vi "CREAR_BANDEJA_xml.vi"(0 "largo":u32, 1 "nombre bandeja":string, 2 "Nº de filas":u32, 3 "Nº de columnas":u32, 4 "Paso X":dbl, 5 "error in (no error)":errorcluster, 6 "path":path, 7 "Paso Y":dbl, 9 "DISTANCIA SUELO A CHIP":dbl, 10 "ancho":u32, 11 "Dist. borde bandeja a centro chip":dbl) -> (19 "error out":errorcluster)   [LabVIEW 2019]
uses:
  <vilib>/Utility/error.llb/Error Cluster From Error Code.vi
  <vilib>/Utility/xml.llb/Write to XML File(string).vi
  <vilib>/ErrorRing/Error Ring.xnode
panel:
  out "Cluster to XML file":T1
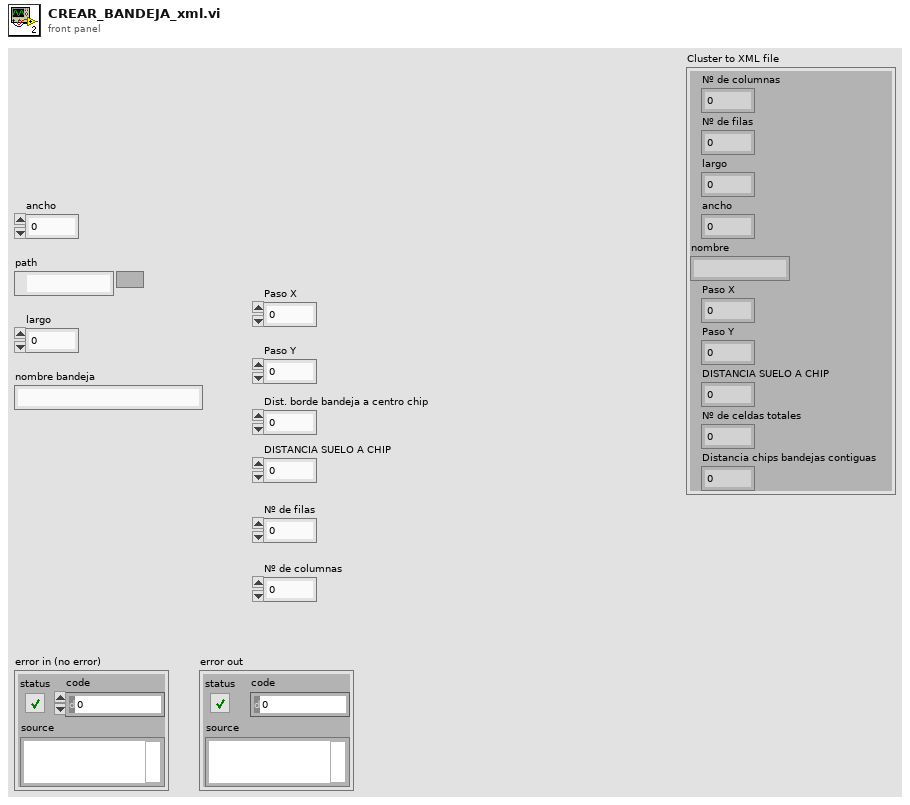
[diagram p1: front panel]
types:
  T1 = cluster{"Nº de columnas ":u16, "Nº de filas ":u16, "largo":u32, "ancho":u32, "nombre":string, "Paso X":dbl, "Paso Y":dbl, "DISTANCIA SUELO A CHIP  ":dbl, "Nº de celdas totales":u16, "Distancia chips bandejas contiguas":dbl}
  T2 = cluster{"Nº de columnas ":u32, "Nº de filas ":u32, "largo":u32, "ancho":u32, "nombre":string, "Paso X":dbl, "Paso Y":dbl, "DISTANCIA SUELO A CHIP  ":dbl, "Nº de celdas totales":u16, "Distancia chips bandejas contiguas":dbl}
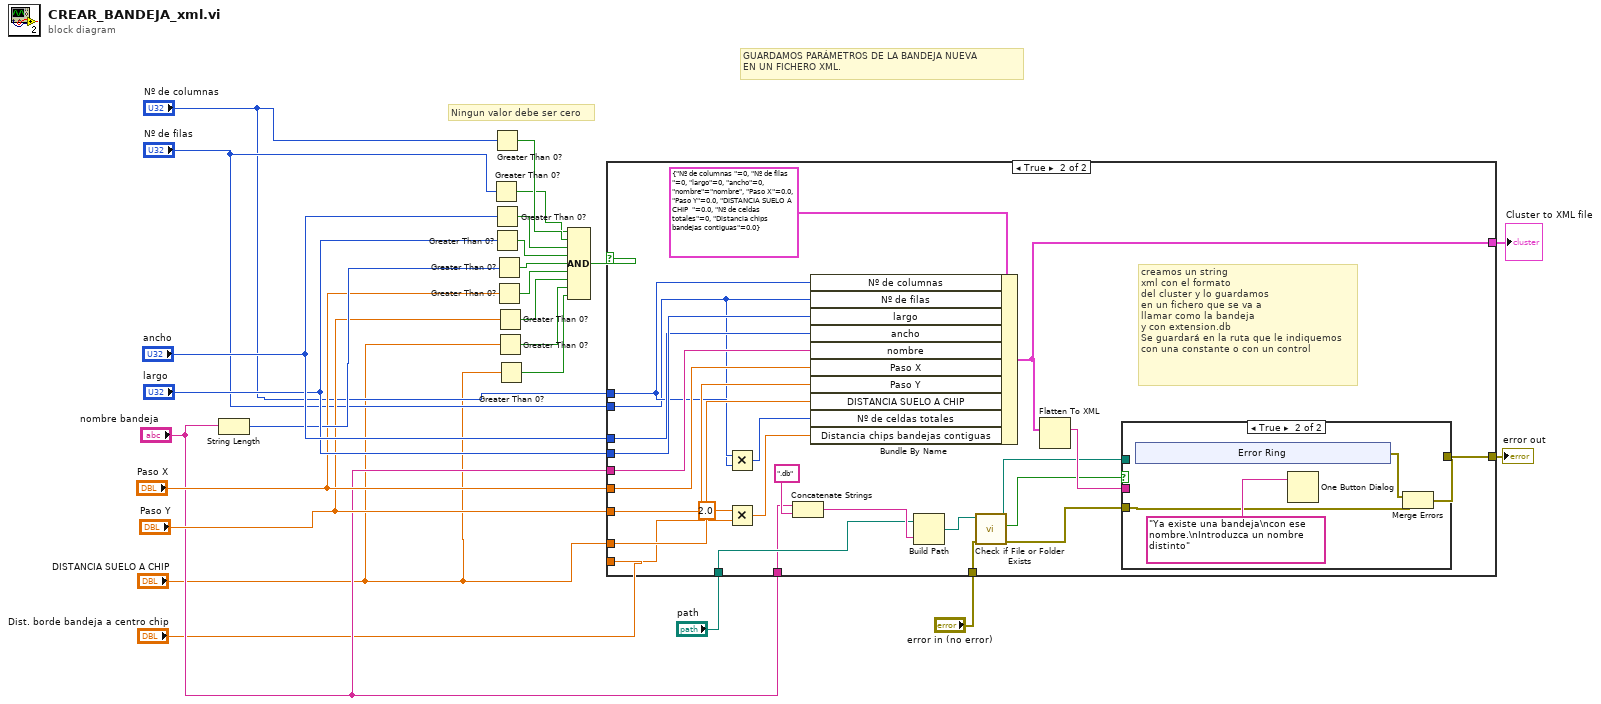
[diagram p0: block diagram]
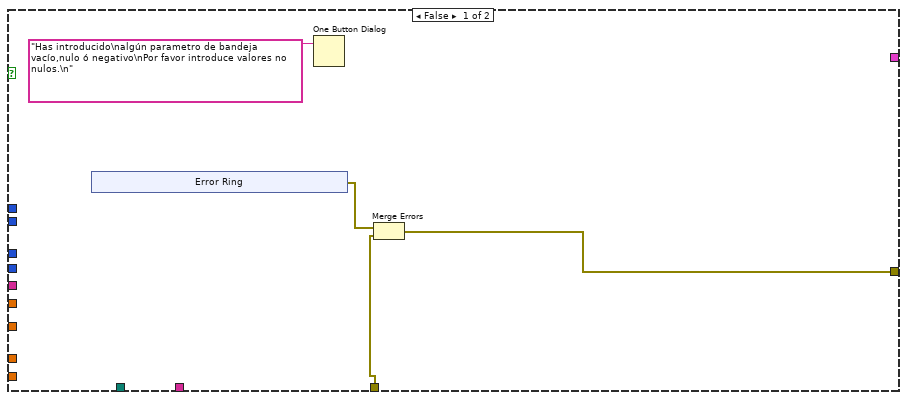
[diagram p2: hidden frame]
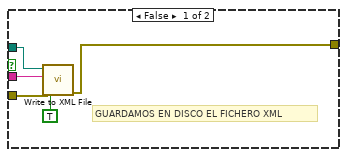
[diagram p3: hidden frame]
diagram:
  # "GUARDAMOS PARÁMETROS DE LA BANDEJA NUEVA\nEN UN FICHERO XML."
  # "Ningun valor debe ser cero"
  n1 = String Length(string="nombre bandeja") -> (length=w18:i32)
  n2 = Greater Than 0?(x="Nº de filas") -> (x > 0?=w6:bool)
  n3 = Greater Than 0?(x="Nº de columnas") -> (x > 0?=w8:bool)
  n4 = Greater Than 0?(x="ancho") -> (x > 0?=w21:bool)
  n5 = Greater Than 0?(x="largo") -> (x > 0?=w22:bool)
  n6 = Greater Than 0?(x=w18) -> (x > 0?=w23:bool)
  n7 = Greater Than 0?(x="Paso X") -> (x > 0?=w14:bool)
  n8 = Greater Than 0?(x="Paso Y") -> (x > 0?=w13:bool)
  n9 = Greater Than 0?(x="DISTANCIA SUELO A CHIP") -> (x > 0?=w7:bool)
  n10 = Greater Than 0?(x="DISTANCIA SUELO A CHIP") -> (x > 0?=w1:bool)
  n11 = Compound Arithmetic op=AND(w6, w8, w21, w22, w23, w14, w13, w7, w1) -> (w24:bool)
  n12 = case shown="True" w24 {
    tunnel: "path" -> [_ w55]
    tunnel: "ancho" -> [_ w47]
    tunnel: "largo" -> [_ w48]
    tunnel: "nombre bandeja" -> [_ w54]
    tunnel: "nombre bandeja" -> [_ w46]
    tunnel: "Paso X" -> [_ w45]
    tunnel: "Paso Y" -> [_ w44]
    tunnel: [w26 w53] -> w12
    tunnel: "Nº de filas" -> [_ w38]
    tunnel: "Nº de columnas" -> [_ w39]
    tunnel: "DISTANCIA SUELO A CHIP" -> [_ w43]
    tunnel: [_ w42] -> w3
    tunnel: "error in (no error)" -> [w25 w41]
    tunnel: "Dist. borde bandeja a centro chip" -> [_ w36]
    frame False {
      n13 = xnode "Error Ring"() -> ("error out"=w27:errorcluster)
      n14 = One Button Dialog(message="Has introducido\nalgún parametro de bandeja vacío,nulo ó negativo\nPor favor introduce valores no nulos.\n") -> ()  [unwired: 1 in, 1 out]
      n15 = Merge Errors(w27, w25) -> (w26:errorcluster)
    }
    frame True {
      # "creamos un string\nxml con el formato\ndel cluster y lo guardamos\nen un fichero que se va a\nllamar como la bandeja\ny con extension.db\nSe guardará en la ruta que le indiquemos\ncon una constante o con un control"
      n16 = Multiply(x=w39, y=w38) -> (x*y=w37:u32)
      n17 = Multiply(x=2.0, y=w36) -> (x*y=w34:dbl)
      n18 = Concatenate Strings(w54, ".db" ("string")) -> (w56:string)
      n19 = Bundle By Name(cluster=T2 {"Nº de columnas "=0, "Nº de filas "=0, "largo"=0, "ancho"=0, "nombre"="nombre", "Paso X"=0.0, "Paso Y"=0.0, "DISTANCIA SUELO A CHIP  "=0.0, "Nº de celdas totales"=0, "Distancia chips bandejas contiguas"=0.0}, "Nº de columnas"=w39, "Nº de filas"=w38, "largo"=w48, "ancho"=w47, "nombre"=w46, "Paso X"=w45, "Paso Y"=w44, "DISTANCIA SUELO A CHIP"=w43, "Nº de celdas totales"=w37, "Distancia chips bandejas contiguas"=w34) -> (w42:T2)
      n20 = Build Path(base path=w55, name or relative path=w56) -> (appended path=w52:path)
      n21 = call <vilib>:"Check if File or Folder Exists.vi"("error in (no error)"=w41, "path"=w52) -> ("error out"=w40:errorcluster, "file or folder exists?"=w51:bool, "dup path"=w50:path)  [unwired: 7 in]
      n22 = Flatten To XML(anything=w42) -> (xml string=w58:string)
      n23 = case shown="True" w51 {
        tunnel: w58 -> [w63 _]
        tunnel: [w61 w65] -> w53
        tunnel: w50 -> [w60 _]
        tunnel: w40 -> [w59 w64]
        frame False {
          # "GUARDAMOS EN DISCO EL FICHERO XML"
          n24 = call-poly <vilib>:"Write to XML File.vi"("Standalone? (T)"=TRUE, "error in (no error)"=w59, "XML Input"=w63, "XML File Path"=w60) -> ("error out"=w61:errorcluster)  [unwired: 5 in, 2 out]
        }
        frame True {
          n25 = xnode "Error Ring"() -> ("error out"=w66:errorcluster)
          n26 = One Button Dialog(message="Ya existe una bandeja\ncon ese nombre.\nIntroduzca un nombre distinto") -> ()  [unwired: 1 in, 1 out]
          n27 = Merge Errors(w66, w64) -> (w65:errorcluster)
        }
      }
    }
  }
  "error out" <- w12
  "Cluster to XML file" <- w3
